vi "Part 1.vi"(11 "Input":string) -> (3 "Output":i64)   [LabVIEW 2021]
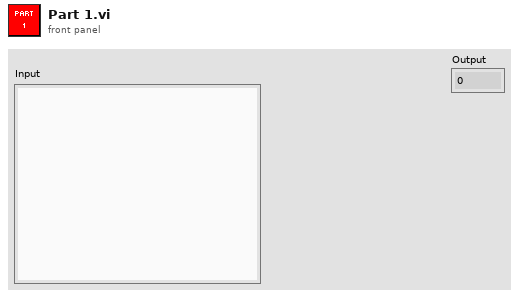
[diagram p1: front panel]
types:
  T1 = cluster{"X Min":i64, "X Max":i64, "Y Min":i64, "Y Max":i64, "Z Min":i64, "Z Max":i64}
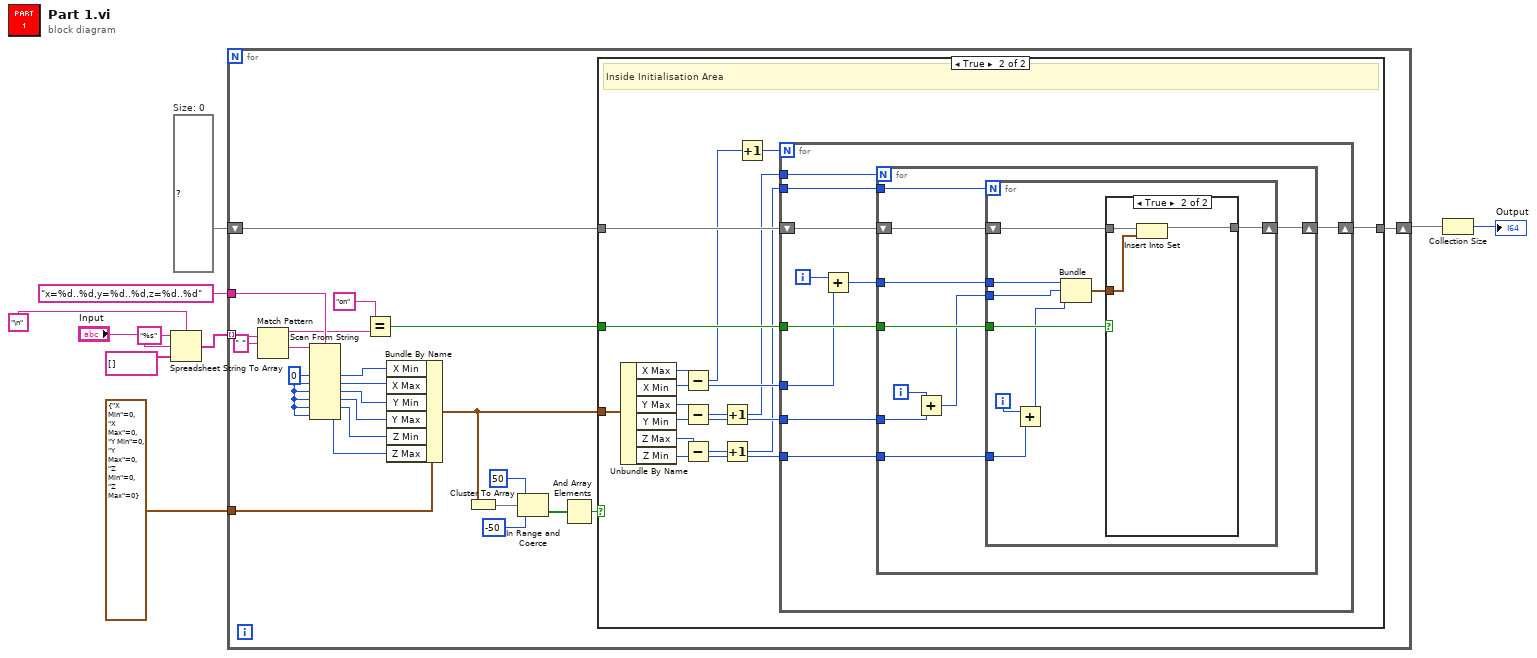
[diagram p0: block diagram]
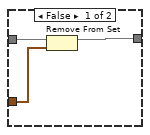
[diagram p3: hidden frame]
diagram:
  w8 = set{cluster{"X":i64, "Y":i64, "Z":i64}} {}  # Size: 0
  n1 = Spreadsheet String To Array(delimiter (Tab)="\n", format string="%s", spreadsheet string="Input", array type (2D Dbl)=string[] []) -> (array=w10:string[])
  n2 = for {
    tunnel: w10 -> [w33] mode=indexing
    tunnel: "x=%d..%d,y=%d..%d,z=%d..%d" ("format string") -> [w31]
    shift-right: [w15] -> w7
    shift-left: w8 -> [w16]
    tunnel: T1 {"X Min"=0, "X Max"=0, "Y Min"=0, "Y Max"=0, "Z Min"=0, "Z Max"=0} -> [w13]
    w22 = i64 0 ("default value 1")
    n3 = Match Pattern(string=w33, regular expression=" ") -> (before substring=w30:string, after substring=w32:string)  [unwired: 1 in, 2 out]
    n4 = Scan From String(format string=w31, input string=w32, default 1=w22, default 2=w22, default 3=w22, default 4=w22, default 5=w22, default 6=w22) -> (output 1=w28:i64, output 2=w27:i64, output 3=w26:i64, output 4=w25:i64, output 5=w24:i64, output 6=w23:i64)  [unwired: 2 in, 3 out]
    n5 = Equal?(x="on", y=w30) -> (x = y?=w14:bool)
    n6 = Bundle By Name(cluster=w13, "X Min"=w28, "X Max"=w27, "Y Min"=w26, "Y Max"=w25, "Z Min"=w24, "Z Max"=w23) -> (w12:T1)
    n7 = Cluster To Array(cluster=w12) -> (array=w21:i64[])
    n8 = In Range and Coerce(upper limit=i64 50, x=w21, lower limit=i64 -50) -> (In Range?=w18:bool[])  [unwired: 1 out]
    n9 = And Array Elements(Boolean array=w18) -> (logical AND=w17:bool)
    n10 = case shown="True" w17 {
      tunnel: w16 -> [w34 w49]
      tunnel: [w34 w48] -> w15
      tunnel: w14 -> [_ w50]
      tunnel: w12 -> [_ w47]
      frame False {
        # "Outside Initialisation Area"
      }
      frame True {
        # "Inside Initialisation Area"
        n11 = Unbundle By Name(w47) -> ("X Max"=w46:i64, "X Min"=w43:i64, "Y Max"=w42:i64, "Y Min"=w39:i64, "Z Max"=w37:i64, "Z Min"=w35:i64)
        n12 = Subtract(x=w46, y=w43) -> (x-y=w45:i64)
        n13 = Subtract(x=w42, y=w39) -> (x-y=w41:i64)
        n14 = Subtract(x=w37, y=w35) -> (x-y=w38:i64)
        n15 = Increment(x=w41) -> (x+1=w40:i64)
        n16 = Increment(x=w38) -> (x+1=w36:i64)
        n17 = Increment(x=w45) -> (x+1=w44:i64)
        n18 = for {
          N: w44 -> [_]
          tunnel: w50 -> [w60]
          shift-right: [w58] -> w48
          shift-left: w49 -> [w59]
          tunnel: w43 -> [w55]
          tunnel: w40 -> [w54]
          tunnel: w39 -> [w53]
          tunnel: w36 -> [w52]
          tunnel: w35 -> [w51]
          i -> [w57]
          n19 = Add(x=w57, y=w55) -> (x+y=w56:i64)
          n20 = for {
            N: w54 -> [_]
            tunnel: w60 -> [w69]
            tunnel: w56 -> [w66]
            shift-right: [w67] -> w58
            shift-left: w59 -> [w68]
            tunnel: w53 -> [w65]
            tunnel: w52 -> [w62]
            tunnel: w51 -> [w61]
            i -> [w64]
            n21 = Add(x=w64, y=w65) -> (x+y=w63:i64)
            n22 = for {
              N: w62 -> [_]
              tunnel: w69 -> [w78]
              tunnel: w66 -> [w73]
              tunnel: w63 -> [w72]
              shift-right: [w76] -> w67
              shift-left: w68 -> [w77]
              tunnel: w61 -> [w74]
              i -> [w75]
              n23 = Add(x=w75, y=w74) -> (x+y=w71:i64)
              n24 = Bundle(w73, w72, w71) -> (w70:cluster{i64, i64, i64})  [unwired: 1 in]
              n25 = case shown="True" w78 {
                tunnel: w77 -> [w80 w84]
                tunnel: [w81 w83] -> w76
                tunnel: w70 -> [w79 w82]
                frame False {
                  n26 = Remove From Set(10:w79, 11:w80) -> (3:w81:set{cluster{"X":i64, "Y":i64, "Z":i64}})  [unwired: 1 out]
                }
                frame True {
                  n27 = Insert Into Set(10:w82, 11:w84) -> (3:w83:set{cluster{"X":i64, "Y":i64, "Z":i64}})  [unwired: 1 out]
                }
              }
            }
          }
        }
      }
    }
  }
  n28 = Collection Size(1:w7) -> (0:→"Output":i32)
